vi "Test Cal.vi"() -> ()   [LabVIEW 2024]
panel:
  in  "Numeric":dbl
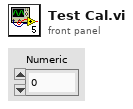
[diagram p1: front panel]
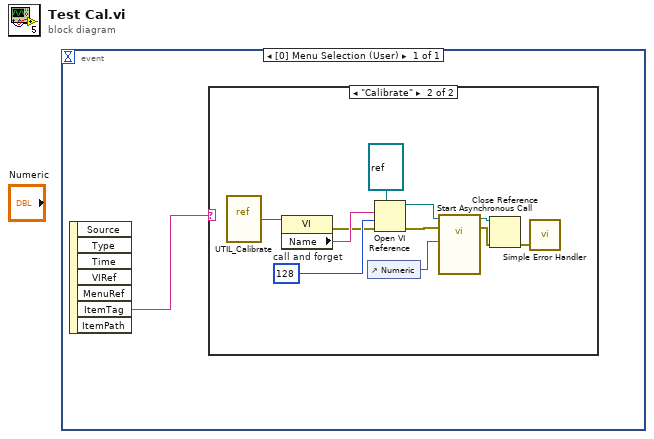
[diagram p0: block diagram]
diagram:
  n1 = event shown="[0] Menu Selection (User)" {
    selector: _ -> [_]
    dyn-events: _ -> [_]
    timeout: _ -> [_]
    event Menu Selection (User) {
      n2 = event-data() -> ("ItemTag"=w1:string)  [unwired: 1 in, 6 out]
      n3 = case shown="\"Calibrate\"" w1 {
        frame "False", Default {
        }
        frame "Calibrate" {
          w12 = 128  # call and forget
          n4 = vi-ref "UTIL_Calibrate.vi"() -> (w5:refnum<vi>)
          n5 = property class="VI"(reference=w5) -> (error out=w3:errorcluster, "Name"=w4:string)  [unwired: 1 in, 1 out]
          n6 = control-ref of="Numeric"() -> (w2:refnum<vi>)
          n7 = Open VI Reference(type specifier VI Refnum (for type only)=refnum<vi> refnum, vi path=w4, options=w12, error in (no error)=w3) -> (vi reference=w10:refnum<vi>, error out=w9:errorcluster)  [unwired: 2 in]
          n8 = call-by-ref "Start Asynchronous Call"(reference=w10, error in=w9, "Digital in"=w2) -> (reference out=w7:refnum<vi>, error out=w8:errorcluster)  [unwired: 10 in, 1 out]
          n9 = Close Reference(reference=w7, error in (no error)=w8) -> (error out=w6:errorcluster)
          n10 = call <vilib>:"Simple Error Handler.vi"("error in (no error)"=w6) -> ()  [unwired: 4 in, 5 out]
        }
      }
    }
  }
